vi "construct.vi"(8 "error in (no error)":errorcluster, 11 "DAQ  in":refnum<class "DAQ .lvclass">) -> (0 "error out":errorcluster, 3 "DAQ  out":refnum<class "DAQ .lvclass">)   [LabVIEW 2016, in "Hardware.lvlib" / "DAQ .lvclass"]
uses:
  DAQ .lvclass
  \\Mac\Home/Documents/MAL-Framework/user.lib/Common Components/Hardware/Hardware.lvclass
  config/DAQ Configuration.lvclass
  \\Mac\Home/Documents/MAL-Framework/user.lib/Common Components/Hardware/HW Config/HW Configuration.lvclass
  Hardware.lvclass/Hardware.ctl
  Hardware.lvclass
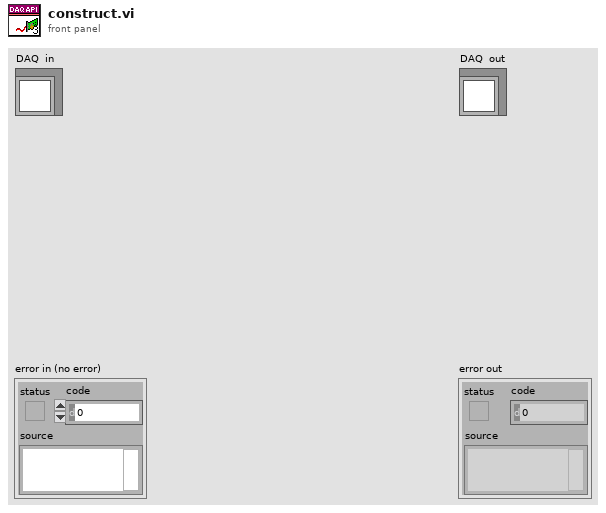
[diagram p1: front panel]
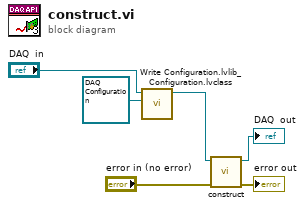
[diagram p0: block diagram]
diagram:
  n1 = call "Write Configuration.lvlib_Configuration.lvclass.vi"("Hardware.lvlib:HW Configuration.lvclass"=refnum<class "DAQ Configuration.lvclass"> refnum ("Hardware.lvlib:DAQ Configuration.lvclass"), "Hardware in"="DAQ  in") -> ("Hardware out"=w2:refnum<class "DAQ .lvclass">)  [unwired: 8 in, 1 out]
  n2 = call-parent "construct.vi"("error in (no error)"="error in (no error)", "Hardware in"=w2) -> ("error out"=→"error out":errorcluster, "Hardware out"=→"DAQ  out":refnum<class "DAQ .lvclass">)  [unwired: 8 in]
